vi "ma_SML RT Zoom FFT Power Spectrum (real input).vi"(4 "master reset?":bool, 6 "reset averaging?":bool, 7 "averaging parameters":T1={"averaging type"=enum."no averaging", "averaging settings"={"weighting type"=enum."linear", "weighting settings"={"size"=10.0, "linear weighting mode"=enum."moving average"}}}, 8 "error in (no error)":errorcluster, 9 "zoom FFT settings":T3={"zoom settings"={"center frequency"=-inf, "zoom"=1, "trim"=1.0}, "FFT settings"={"window"=1, "window size"=-1, "FFT size"=1024, "%overlap"=0.0}} {"FFT settings"."%overlap" min=0.0 max=100.0 format="%.2f"; "FFT settings"."window" items=["Rectangle"=0, "Hanning"=1, "Hamming"=2, "Blackman-Harris"=3, "Exact Blackman"=4, "Blackman"=5, "Flat Top"=6, "4 Term B-Harris "=7, "7 Term B-Harris"=8, "Low Sidelobe"=9, "Blackman Nuttall"=11, "Triangle"=30, "Bartlett-Hanning"=31, "Bohman"=32, "Parzen"=33, "Welch"=34, "Kaiser"=60, "Dolph-Chebyshev"=61, "Gaussian"=62]; "zoom settings"."trim" min=1.0 format="%.2f"; "zoom settings"."center frequency" format="%.2f"; "zoom settings"."zoom" min=1}, 10 "fs":dbl=1024.0 format="%.2f", 11 "x":dbl[](array[numeric]) format="%.2f") -> (0 "error out":errorcluster, 1 "data ready?":bool, 2 "spectral info":T5 {"window" items=["Rectangle"=0, "Hanning"=1, "Hamming"=2, "Blackman-Harris"=3, "Exact Blackman"=4, "Blackman"=5, "Flat Top"=6, "4 Term B-Harris "=7, "7 Term B-Harris"=8, "Low Sidelobe"=9, "Blackman Nuttall"=11, "Triangle"=30, "Bartlett-Hanning"=31, "Bohman"=32, "Parzen"=33, "Welch"=34, "Kaiser"=60, "Dolph-Chebyshev"=61, "Gaussian"=62]}, 3 "power spectrum":T4={"f0"=0.0, "df"=1.0, "spectrum"=[]} {"spectrum" format="%.2f"; "df" format="%.2f"; "f0" format="%.2f"}, 5 "averaged sofar":dbl)   [LabVIEW 2020, in "NI_MAPro.lvlib"]
uses:
  NI_MAPro.lvlib
  ma_sml_Spectral Info.ctl
  ma_sml_Spectrum Cluster (real).ctl
  ma_sml_RT Zoom FFT Settings.ctl
  ma_sml_Averaging Parameters.ctl
  ma_sml_Averaging Settings.ctl
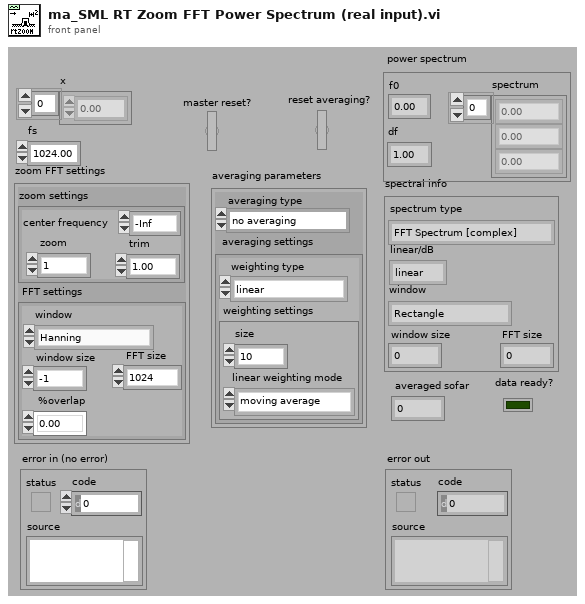
[diagram p1: front panel]
types:
  T1 = typedef "NI_MAPro.lvlib/ma_sml_Averaging Parameters.ctl" = cluster{"averaging type":enum16{"no averaging", "vector averaging", "RMS averaging", "peak hold"}, "averaging settings":T2}
  T2 = typedef "NI_MAPro.lvlib/ma_sml_Averaging Settings.ctl" = cluster{"weighting type":enum16{"linear", "exponential"}, "weighting settings":cluster{"size":dbl, "linear weighting mode":enum16{"one shot", "auto restart one shot", "moving average", "continuous"}}}
  T3 = typedef "NI_MAPro.lvlib/ma_sml_RT Zoom FFT Settings.ctl" = cluster{"zoom settings":cluster{"center frequency":dbl, "zoom":i32, "trim":dbl}, "FFT settings":cluster{"window":u16, "window size":i32, "FFT size":i32, "%overlap":dbl}}
  T4 = typedef "NI_MAPro.lvlib/ma_sml_Spectrum Cluster (real).ctl" = cluster{"f0":dbl, "df":dbl, "spectrum":dbl[]}
  T5 = typedef "NI_MAPro.lvlib/ma_sml_Spectral Info.ctl" = cluster{"spectrum type":enum16{"FFT Spectrum [complex]", "Amplitude [Magnitude]", "Power [Magnitude^2]", "Cross Spectrum [complex]", "Frequency Response [Complex]"}, "linear/dB":enum16{"linear", "dB"}, "window":u16, "window size":i32, "FFT size":i32}
  T6 = typedef "NI_MAPro.lvlib/ma_sml_Spectrum Cluster (complex).ctl" = cluster{"f0":dbl, "df":dbl, "spectrum":cdb[]}
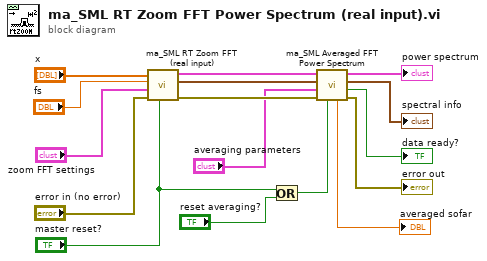
[diagram p0: block diagram]
diagram:
  n1 = call "ma_SML RT Zoom FFT (real input).vi"("reset?"="master reset?", "error in (no error)"="error in (no error)", "zoom FFT settings"="zoom FFT settings", "fs"="fs", "x"="x") -> ("error out"=w15:errorcluster, "spectral info"=w8:T5, "FFT spectrum"=w9:T6)  [unwired: 2 in, 2 out]
  n2 = Or(x="master reset?", y="reset averaging?") -> (x .or. y?=w12:bool)
  n3 = call "ma_SML Averaged FFT Power Spectrum.vi"("reset averaging?"=w12, "error in (no error)"=w15, "averaging parameters"="averaging parameters", "spectral info in"=w8, "FFT spectrum"=w9) -> ("error out"=→"error out":errorcluster, "data ready?"=→"data ready?":bool, "spectral info out"=→"spectral info":T5, "avg power spectrum"=→"power spectrum":T4, "averages sofar"=→"averaged sofar":dbl)  [unwired: 2 out]
